vi "doAction.vi"(0 "HGF_FGV_Action":refnum<class "HGF_FGV_Action.lvclass">, 2 "Objects":refnum<class>[](array[class]), 5 "error in (no error)":errorcluster) -> (14 "dup HGF_FGV_Action":refnum<class "HGF_FGV_Action.lvclass">, 16 "dup Objects":refnum<class>[](array[class]), 19 "error out":errorcluster)   [LabVIEW 2012, in "HGF_FGV.lvlib" / "HGF_FGV_Action.lvclass"]
doc: "This VI calls the protected dynamic action.vi that can be overwritten by child classes."
uses:
  HGF_FGV_Action.lvclass
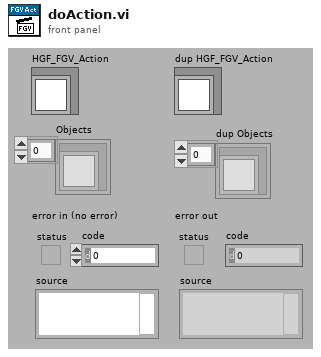
[diagram p1: front panel]
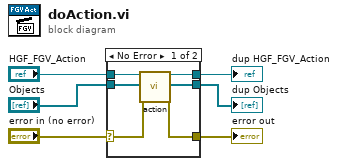
[diagram p0: block diagram]
diagram:
  n1 = case shown="No Error" "error in (no error)" {
    selector: "error in (no error)" -> [w7 w13]
    tunnel: [w11 w15] -> w5
    tunnel: "HGF_FGV_Action" -> [w12 w15]
    tunnel: "Objects" -> [w10 w14]
    tunnel: [w9 w14] -> w2
    tunnel: [w8 w13] -> w1
    frame No Error {
      n2 = call-dynamic "action.vi"("HGF_FGV_Action"=w12, "Objects"=w10, "error in (no error)"=w7) -> ("dup HGF_FGV_Action"=w11:refnum<class "HGF_FGV_Action.lvclass">, "dup Objects"=w9:refnum<class>[], "error out"=w8:errorcluster)  [unwired: 14 out]
    }
    frame Error {
    }
  }
  "error out" <- w1
  "dup HGF_FGV_Action" <- w5
  "dup Objects" <- w2
